vi "DPT Panel Get Final Weight.vi"(7 "Init value(\"\")":string) -> (8 "Final Load  Weight Out":string(combo))   [LabVIEW 2014]
panel:
  in  "Enter Final Load Weight":string
  in  "stop":bool
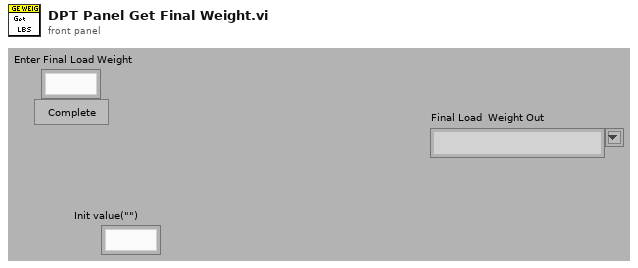
[diagram p1: front panel]
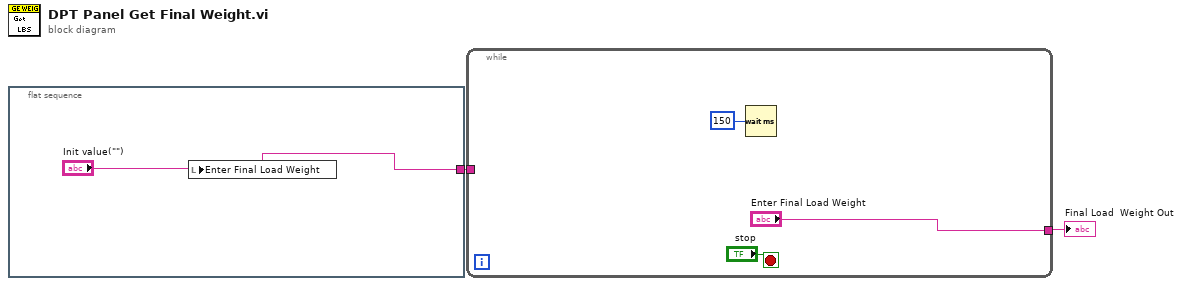
[diagram p0: block diagram]
diagram:
  n1 = flat-sequence {
    tunnel: ["Init value(\"\")"] -> w1
    frame #0 {
      n2 = local write "Enter Final Load Weight"("Init value(\"\")") -> ()
    }
  }
  n3 = while {
    tunnel: ["Enter Final Load Weight"] -> w2
    tunnel: w1 -> [_]
    stop <- "stop" stop-if-true
    n4 = Wait (ms)(milliseconds to wait=u32 150) -> ()  [unwired: 1 out]
  }
  "Final Load  Weight Out" <- w2
